vi "To CSV File.vi"(8 "error in (no error)":errorcluster, 9 "Path":path, 10 "engine configuration":refnum<class "engine configuration.lvclass">, 11 "PID Module 2 editor node in":refnum<class "PID Module 2 editor node.lvclass">) -> (0 "error out":errorcluster, 3 "PID Module 2 editor node out":refnum<class "PID Module 2 editor node.lvclass">)   [LabVIEW 2015, in "PID Module 2 editor node.lvclass"]
uses:
  PID Module 2 editor node.lvclass
  <vilib>/NI/Module Execution Interface/Engine Configuration/engine configuration.lvclass
  module/configuration/PID Module 2 configuration.lvclass
  <vilib>/NI/Configuration Framework/serializable configuration/NISE_CEF_serializable configuration.lvclass/NISE_CEF_serializable configuration.ctl
  module/configuration/PID Module 2 configuration.lvclass/PID Module 2 configuration.ctl
  <vilib>/Utility/LVClass/Get LV Class Name.vi
  <vilib>/NI/Configuration Framework/error generator/NISE_error generator.vi
  <vilib>/NI/Tag Bus Module Framework/channel/TBM channel.lvclass
  <vilib>/NI/Configuration Framework/serializable configuration/NISE_CEF_serializable configuration.lvclass
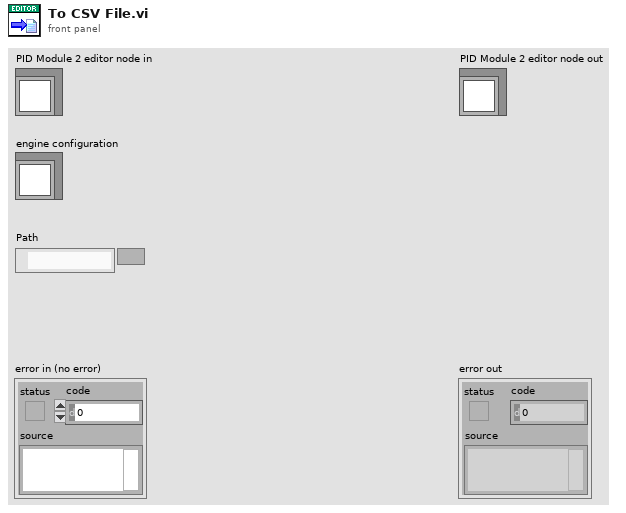
[diagram p1: front panel]
types:
  T1 = typedef "PID Module 2 configuration.lvclass/Line.ctl" = cluster{"PID ID":string, "Setpoint":refnum<class "TBM channel.lvclass">, "Variable":refnum<class "TBM channel.lvclass">, "Output":refnum<class "TBM channel.lvclass">, "Output High":refnum<class "TBM channel.lvclass">, "Output Low":refnum<class "TBM channel.lvclass">, "P":refnum<class "TBM channel.lvclass">, "I":refnum<class "TBM channel.lvclass">, "D":refnum<class "TBM channel.lvclass">}
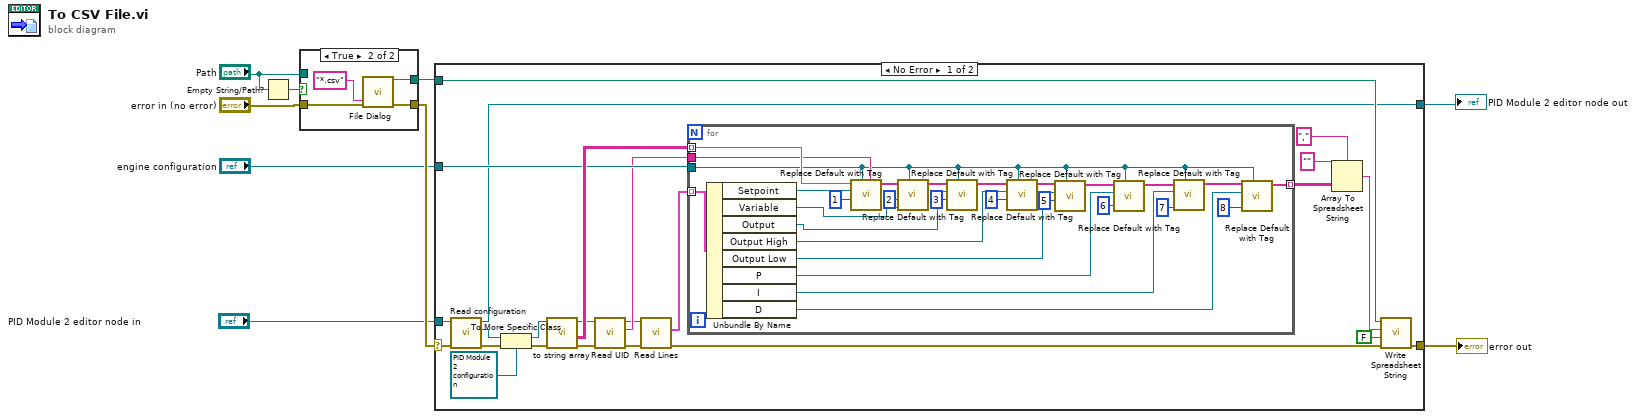
[diagram p0: block diagram]
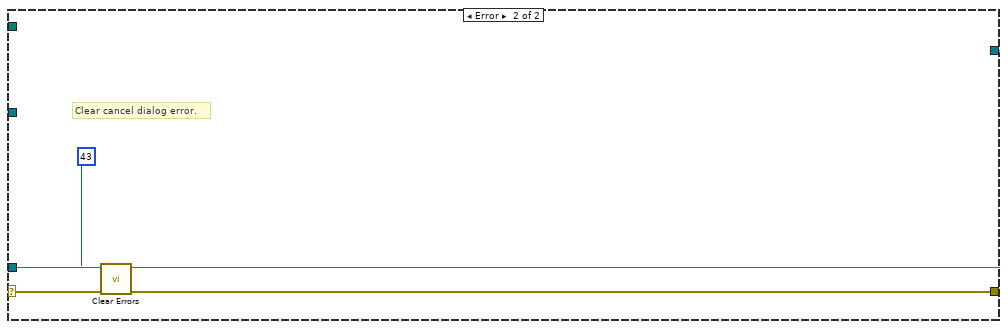
[diagram p3: hidden frame]
diagram:
  n1 = Empty String/Path?(string/path="Path") -> (empty?=w9:bool)
  n2 = case shown="True" w9 {
    tunnel: "error in (no error)" -> [w10 w14]
    tunnel: [w10 w13] -> w7
    tunnel: [w11 w12] -> w8
    tunnel: "Path" -> [w11 _]
    frame False {
    }
    frame True {
      n3 = call "File Dialog"("error in"=w14, "pattern (all files)"="*.csv") -> ("selected path"=w12:path, "error out"=w13:errorcluster)  [unwired: 10 in, 2 out]
    }
  }
  n4 = case shown="No Error" w7 {
    selector: w7 -> [w26 w70]
    tunnel: [w37 w69] -> w2
    tunnel: [w25 w71] -> w1
    tunnel: "PID Module 2 editor node in" -> [w27 w71]
    tunnel: w8 -> [w33 _]
    tunnel: "engine configuration" -> [w30 _]
    frame No Error {
      n5 = call-dynamic "Read configuration.vi"("error in"=w26, "PID Module 2 editor node in"=w27) -> ("error out"=w24:errorcluster, "configuration"=w23:refnum<class "NISE_CEF_serializable configuration.lvclass">, "PID Module 2 editor node out"=w25:refnum<class "PID Module 2 editor node.lvclass">)  [unwired: 7 in]
      n6 = To More Specific Class(target class=refnum<class "PID Module 2 configuration.lvclass"> refnum ("tag bus configurable plugin module configuration"), reference=w23, error in=w24) -> (specific class reference=w39:refnum<class "PID Module 2 configuration.lvclass">, error out=w38:errorcluster)
      n7 = call-dynamic "to string array.vi"("error in (no error)"=w38, "PID Module 2 configuration in"=w39) -> ("error out"=w21:errorcluster, "Array"=w32:string[][], "PID Module 2 configuration out"=w22:refnum<class "PID Module 2 configuration.lvclass">)  [unwired: 6 in, 1 out]
      n8 = call <vilib>:"Read UID.vi"("error in"=w21, "configuration in"=w22) -> ("error out"=w19:errorcluster, "instance id"=w29:string, "configuration out"=w16:refnum<class "PID Module 2 configuration.lvclass">)  [unwired: 7 in]
      n9 = call "Read Lines.vi"("error in (no error)"=w19, "PID Module 2 configuration in"=w16) -> ("error out"=w18:errorcluster, "Lines"=w17:T1[])  [unwired: 7 in, 1 out]
      n10 = for {
        tunnel: w32 -> [w66] mode=indexing
        tunnel: [w53] -> w31 mode=indexing
        tunnel: w17 -> [w67] mode=indexing
        tunnel: w30 -> [w50]
        tunnel: w29 -> [w65]
        n11 = Unbundle By Name(w67) -> ("Setpoint"=w61:refnum<class "TBM channel.lvclass">, "Variable"=w60:refnum<class "TBM channel.lvclass">, "Output"=w59:refnum<class "TBM channel.lvclass">, "Output High"=w58:refnum<class "TBM channel.lvclass">, "Output Low"=w57:refnum<class "TBM channel.lvclass">, "P"=w56:refnum<class "TBM channel.lvclass">, "I"=w52:refnum<class "TBM channel.lvclass">, "D"=w51:refnum<class "TBM channel.lvclass">)
        n12 = call "Replace Default with Tag.vi"("instance id"=w65, "engine configuration in"=w50, "Channel Index"=1, "Channel"=w61, "Array in"=w66) -> ("Array out"=w49:string[])  [unwired: 6 in]
        n13 = call "Replace Default with Tag.vi"("engine configuration in"=w50, "Channel Index"=2, "Channel"=w60, "Array in"=w49) -> ("Array out"=w64:string[])  [unwired: 7 in]
        n14 = call "Replace Default with Tag.vi"("engine configuration in"=w50, "Channel Index"=3, "Channel"=w59, "Array in"=w64) -> ("Array out"=w48:string[])  [unwired: 7 in]
        n15 = call "Replace Default with Tag.vi"("engine configuration in"=w50, "Channel Index"=4, "Channel"=w58, "Array in"=w48) -> ("Array out"=w63:string[])  [unwired: 7 in]
        n16 = call "Replace Default with Tag.vi"("engine configuration in"=w50, "Channel Index"=5, "Channel"=w57, "Array in"=w63) -> ("Array out"=w62:string[])  [unwired: 7 in]
        n17 = call "Replace Default with Tag.vi"("engine configuration in"=w50, "Channel Index"=6, "Channel"=w56, "Array in"=w62) -> ("Array out"=w55:string[])  [unwired: 7 in]
        n18 = call "Replace Default with Tag.vi"("engine configuration in"=w50, "Channel Index"=7, "Channel"=w52, "Array in"=w55) -> ("Array out"=w54:string[])  [unwired: 7 in]
        n19 = call "Replace Default with Tag.vi"("engine configuration in"=w50, "Channel Index"=8, "Channel"=w51, "Array in"=w54) -> ("Array out"=w53:string[])  [unwired: 7 in]
      }
      n20 = Array To Spreadsheet String(delimiter (Tab)=",", array=w31, 3:"" ("format string")) -> (spreadsheet string=w36:string)
      n21 = call <vilib>:"Write Spreadsheet String.vi"("error in"=w18, "append to file? (new file:F)"=FALSE, "spreadsheet string"=w36, "file path (dialog if empty)"=w33) -> ("error out"=w37:errorcluster)  [unwired: 6 in, 1 out]
    }
    frame Error {
      # "Clear cancel dialog error."
      n22 = call <vilib>:"Clear Errors.vi"("error in (no error)"=w70, "specific error code to clear (0: all)"=43) -> ("error out"=w69:errorcluster)  [unwired: 4 in, 1 out]
    }
  }
  "error out" <- w2
  "PID Module 2 editor node out" <- w1
